vi "Abort Acquisition.vi"(8 "Error In":errorcluster, 11 "CCDCamera.lvclass":refnum<class "CCDCamera.lvclass">) -> (0 "Error Out":errorcluster, 3 "CCDCamera.lvclass":refnum<class "CCDCamera.lvclass">)   [LabVIEW 2018, in "CCDCamera.lvclass"]
doc: "This VI aborts the current acquisition."
uses:
  CCDCamera.lvclass
  <userlib>/atmcd32d.llb/Error Code Enum typedef.ctl
  CCDCamera.lvclass/CCDCamera.ctl
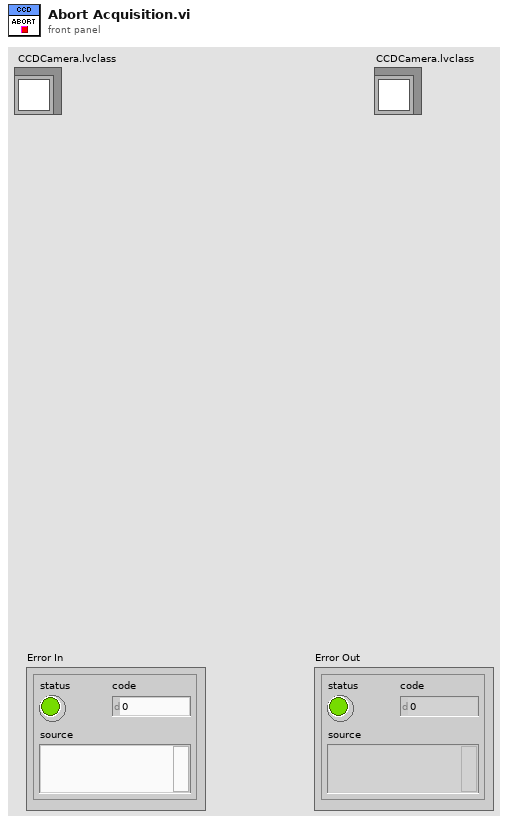
[diagram p1: front panel]
types:
  T1 = typedef "Error Code Enum typedef.ctl" = enum32{"N/A (0)", "DRV_ERROR_CODES", "DRV_SUCCESS", "DRV_VXDNOTINSTALLED", "DRV_ERROR_SCAN", "DRV_ERROR_CHECK_SUM", "DRV_ERROR_FILELOAD", "DRV_UNKNOWN_FUNC", "DRV_ERROR_VXD_INIT", "DRV_ERROR_ADDRESS", "DRV_ERROR_PAGELOCK", "DRV_ERROR_PAGEUNLOCK", "DRV_ERROR_BOARDTEST", "DRV_ERROR_ACK", "DRV_ERROR_UP_FIFO", "DRV_ERROR_PATTERN", "N/A (16)", "DRV_ACQUISITION_ERRORS", "DRV_ACQ_BUFFER", "DRV_ACQ_DOWNFIFO_FULL", "DRV_PROC_UNKONWN_INSTRUCTION", "DRV_ILLEGAL_OP_CODE", "DRV_KINETIC_TIME_NOT_MET", "DRV_ACCUM_TIME_NOT_MET", "DRV_NO_NEW_DATA", "N/A (25)", "DRV_SPOOLERROR", "N/A (27)", "N/A (28)", "N/A (29)", "N/A (30)", "N/A (31)", "N/A (32)", "DRV_TEMPERATURE_CODES", "DRV_TEMPERATURE_OFF", "DRV_TEMPERATURE_NOT_STABILIZED", "DRV_TEMPERATURE_STABILIZED", "DRV_TEMPERATURE_NOT_REACHED", "DRV_TEMPERATURE_OUT_RANGE", "DRV_TEMPERATURE_NOT_SUPPORTED", "DRV_TEMPERATURE_DRIFT", "N/A (41)", "N/A (42)", "N/A (43)", "N/A (44)", "N/A (45)", "N/A (46)", "N/A (47)", "N/A (48)", "DRV_GENERAL_ERRORS", "DRV_INVALID_AUX", "DRV_COF_NOTLOADED", "DRV_FPGAPROG", "DRV_FLEXERROR", "DRV_GPIBERROR", "N/A (55)", "N/A (56)", "N/A (57)", "N/A (58)", "N/A (59)", "N/A (60)", "N/A (61)", "N/A (62)", "N/A (63)", "DRV_DATATYPE", "DRV_DRIVER_ERRORS", "DRV_P1INVALID", "DRV_P2INVALID", "DRV_P3INVALID", "DRV_P4INVALID", "DRV_INIERROR", "DRV_COFERROR", "DRV_ACQUIRING", "DRV_IDLE", "DRV_TEMPCYCLE", "DRV_NOT_INITIALIZED", "DRV_P5INVALID", "DRV_P6INVALID", "DRV_INVALID_MODE", "DRV_INVALID_FILTER", "DRV_I2CERRORS", "DRV_I2CDEVNOTFOUND", "DRV_I2CTIMEOUT", "DRV_P7INVALID", "N/A (84)", "N/A (85)", "N/A (86)", "N/A (87)", "N/A (88)", "N/A (89)", "DRV_IOCERROR", "DRV_VRMVERSIONERROR"}
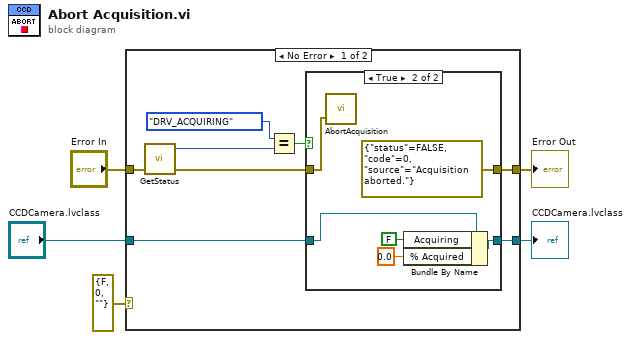
[diagram p0: block diagram]
diagram:
  n1 = case shown="No Error" errorcluster {"status"=FALSE, "code"=0, "source"=""} ("error constant") {
    tunnel: "Error In" -> [w12 w22]
    tunnel: [w13 w22] -> w3
    tunnel: "CCDCamera.lvclass" -> [w7 w23]
    tunnel: [w6 w23] -> w1
    frame No Error {
      n2 = call <userlib>:"GetStatus.vi"("error in (no error)"=w12) -> ("error out"=w8:errorcluster, "status"=w11:T1)  [unwired: 2 in, 1 out]
      n3 = Equal?(x=Error_Code_Enum_typedef."DRV_ACQUIRING", y=w11) -> (x = y?=w9:bool)
      n4 = case shown="True" w9 {
        tunnel: [w15 errorcluster {"status"=FALSE, "code"=0, "source"="Acquisition aborted."} ("error constant")] -> w13
        tunnel: w8 -> [w15 w20]
        tunnel: [w14 w19] -> w6
        tunnel: w7 -> [w14 w18]
        frame False {
        }
        frame True {
          n5 = call <userlib>:"AbortAcquisition.vi"("error in (no error)"=w20) -> ()  [unwired: 1 in, 2 out]
          n6 = Bundle By Name(cluster=w18, "Acquiring"=FALSE, "% Acquired"=0.0) -> (w19:refnum<class "CCDCamera.lvclass">)
        }
      }
    }
    frame Error {
    }
  }
  "CCDCamera.lvclass" <- w1
  "Error Out" <- w3
